vi "Handle Help.vi"(8 "error in (no error)":errorcluster, 10 "Command":variant, 11 "Instrument in":refnum<class "Instrument.lvclass">) -> (0 "error out":errorcluster, 2 "Variant":variant, 3 "Instrument out":refnum<class "Instrument.lvclass">)   [LabVIEW 2019, in "Instrument.lvclass"]
uses:
  Instrument.lvclass
  Typedefs/Instrument.Commands--Enum.ctl
  Typedefs/PrivateEvents--Instrument.DataToLog.ctl
  Typedefs/Instrument.Help--cluster.ctl
  Typedefs/Instrument.API_Help.Param--Cluster.ctl
  5679b731-02d5-469c-8409-12dd10f8f74d.vi
  <vilib>/JDP Science/JSONtext/Variant to JSON Text.vi
  <vilib>/JDP Science/JSONtext/LVClass Serializer/JSONtext LVClass Serializer.lvclass
  <userlib>/LevyLab/JSON-RPC/JSON-RPC.lvlib
  Help/Help.lvclass
  <vilib>/Utility/Data Type/NI_Data Type.lvlib
  <vilib>/JDP Science/JSONtext/JSONtext.lvlib
panel:
  out "<JSON>":string
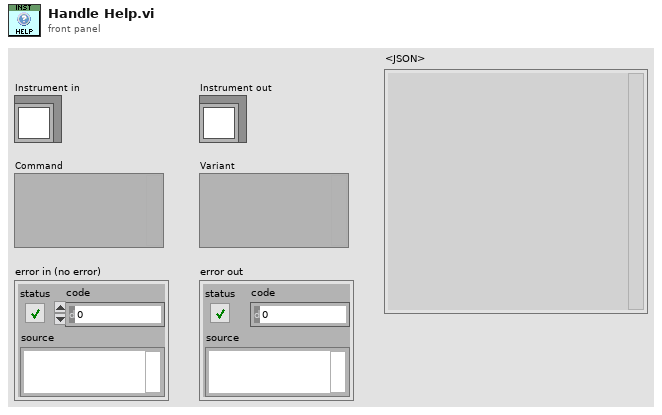
[diagram p1: front panel]
types:
  T1 = typedef "Instrument.lvclass/PrivateEvents--Instrument.DataToLog.ctl" = cluster{"Path(s)":string, "Data":variant}
  T2 = typedef "Instrument.lvclass/Instrument.Commands--Enum.ctl" = enum16{"ACK", "HELP", "setConfiguration", "setLogData", "getAll", "getAllData"}
  T3 = cluster{"number1":dbl, "number2":dbl, "string1":string}
  T4 = typedef "Instrument.lvclass/Instrument.Help--cluster.ctl" = cluster{"description":string, "documentation":string, "example":string}
  T5 = typedef "NI_Data Type.lvlib/Data Type.ctl" = enum8{"Invalid Type", "Void", "I8", "I16", "I32", "I64", "U8", "U16", "U32", "U64", "Single Float", "Double Float", "Extended Float", "Single Complex", "Double Complex", "Extended Complex", "Enum U8", "Enum U16", "Enum U32", "Enum U64", "Single Float With Unit", "Double Float With Unit", "Extended Float With Unit", "Single Complex with Unit", "Double Complex with Unit", "Extended Complex with Unit", "Boolean", "String", "Path", "Picture", "Tag", "Array", "Cluster", "Variant", "LV Variant", "Waveform", "Timestamp", "Digital Waveform", "Digital Data", "ExpressData", "Refnum", "External Data", "VI", "Poly VI", "LabVIEW Class Instance", "Fixed Point", "Set Collection", "Map Collection"}
  T6 = typedef "Instrument.lvclass/Instrument.API_Help.Param--Cluster.ctl" = cluster{"parameter_name":string, "description":string, "min_value":variant, "max_value":variant, "units":string}
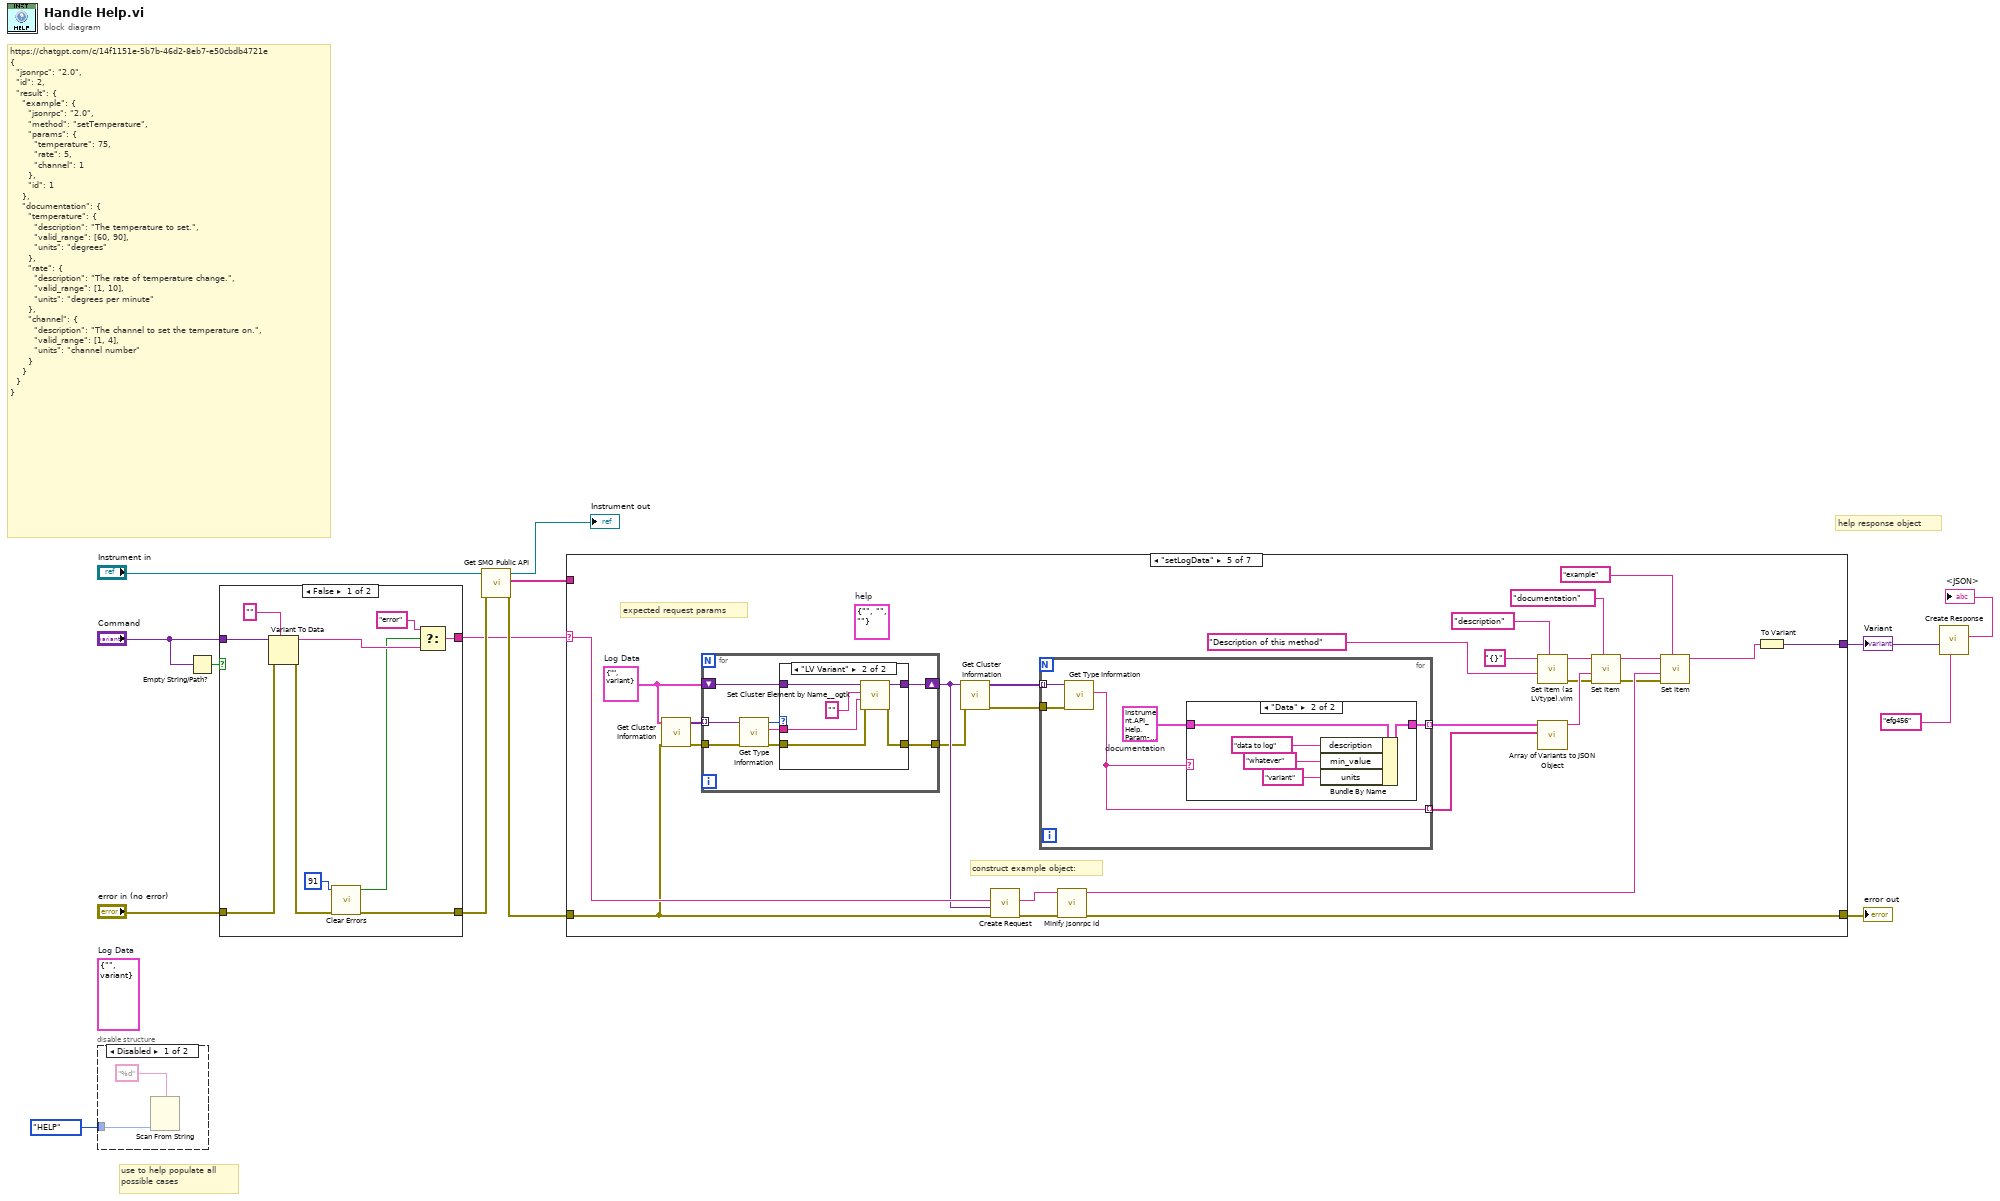
[diagram p0: block diagram]
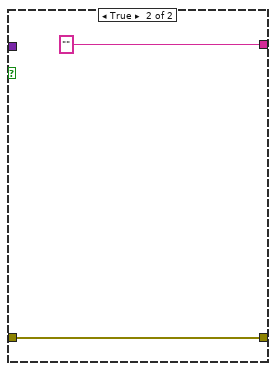
[diagram p2: hidden frame]
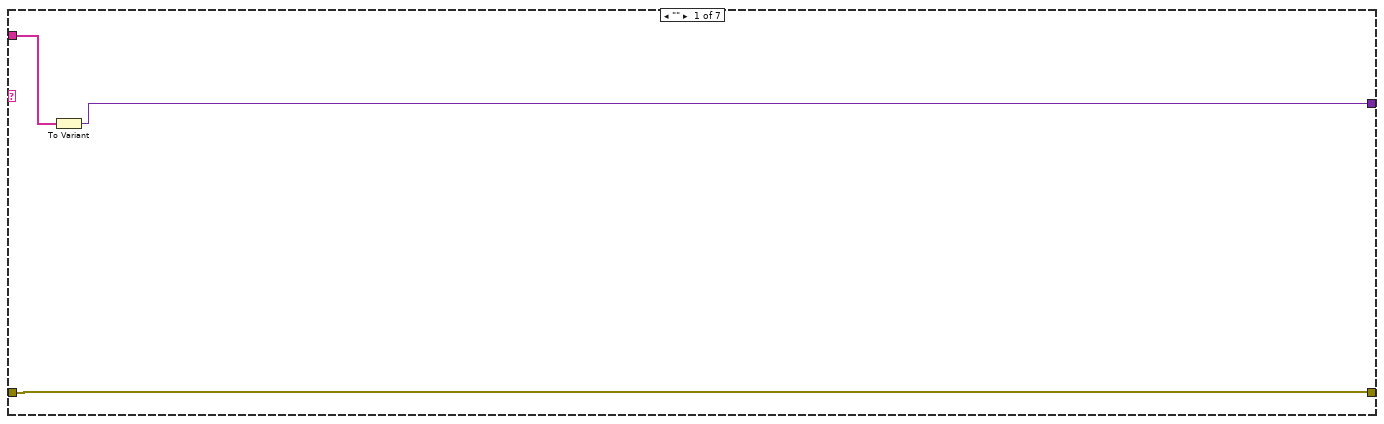
[diagram p4: hidden frame]
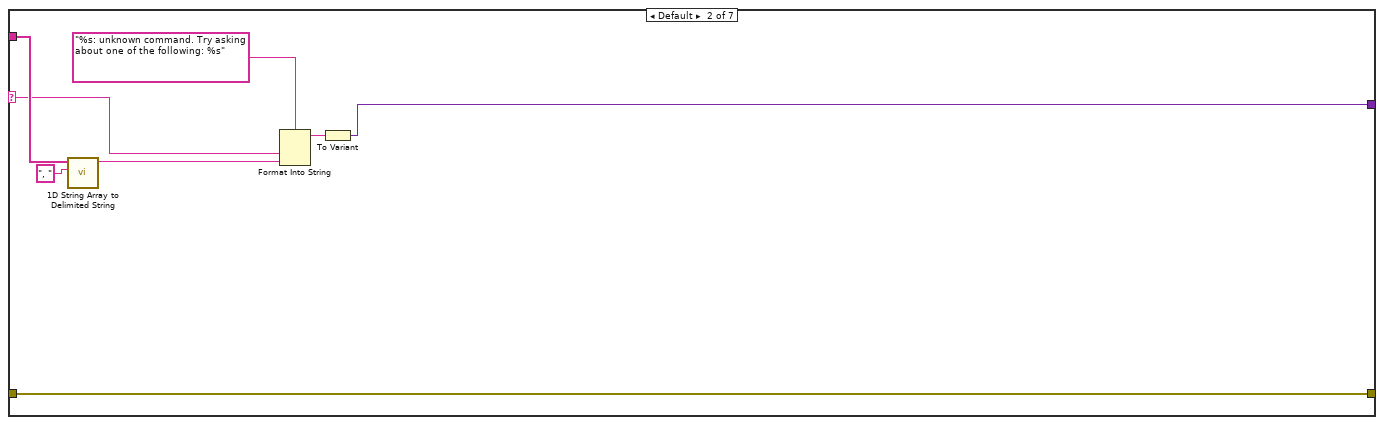
[diagram p5: hidden frame]
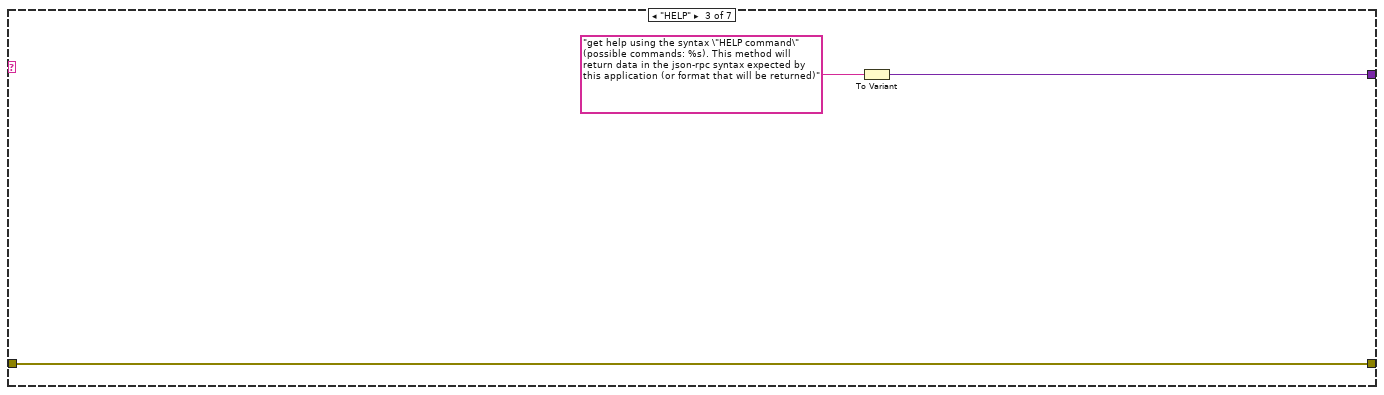
[diagram p6: hidden frame]
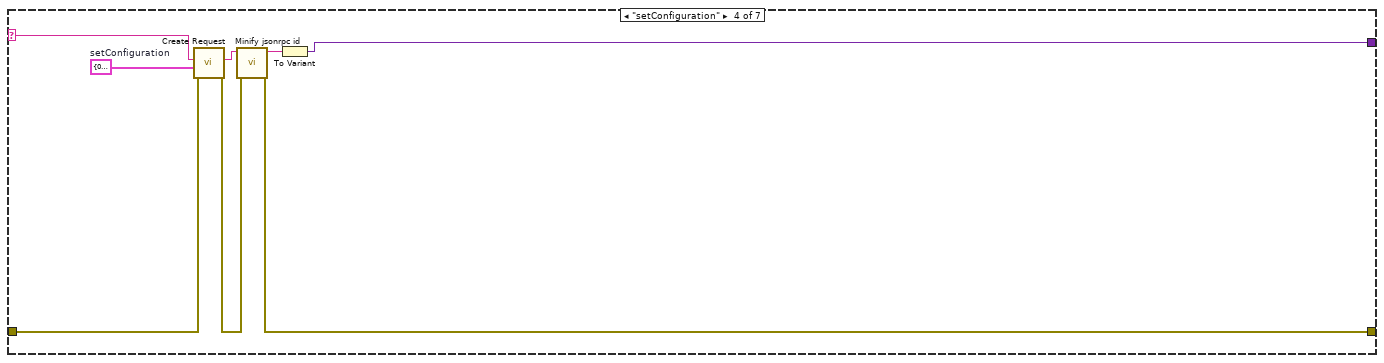
[diagram p7: hidden frame]
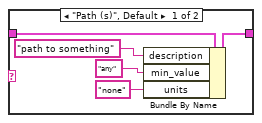
[diagram p9: hidden frame]
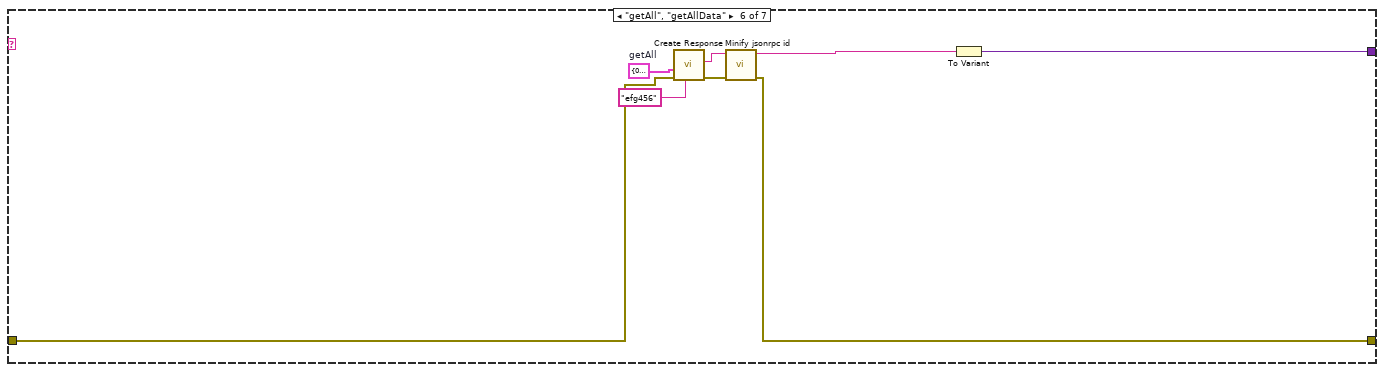
[diagram p10: hidden frame]
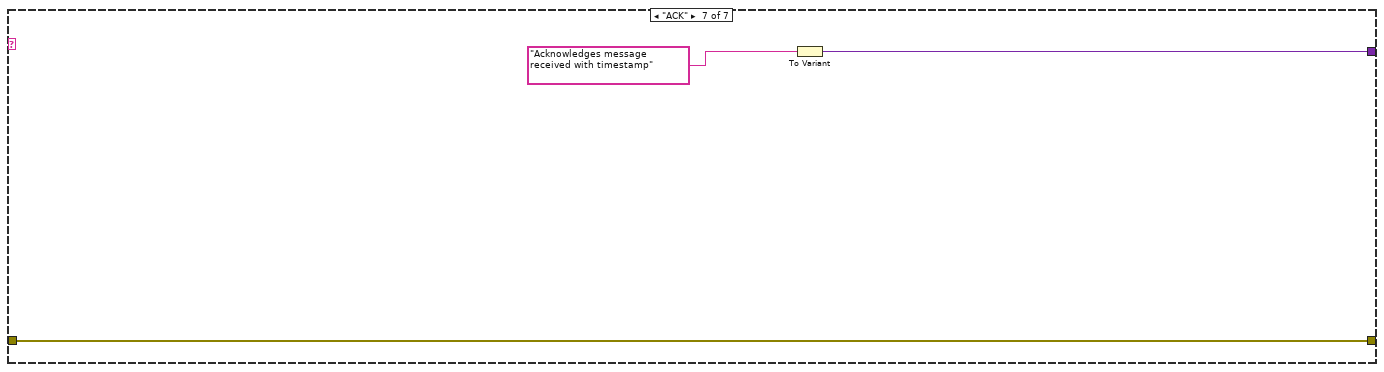
[diagram p11: hidden frame]
diagram:
  (unwired) T1 {"Path(s)"="", "Data"=variant}  # Log Data
  # "help response object"
  # "https://chatgpt.com/c/14f1151e-5b7b-46d2-8eb7-e50cbdb4721e\n{\n  \"jsonrpc\": \"2.0\",\n  \"id\": 2,\n  \"result\": {\n    \"example\": {\n      \"jsonrpc\": \"2.0\",\n      \"method\": \"setTemperature\",\n      \"params\": {\n        \"temperature\": 75,\n        \"rate\": 5,\n        \"channel\": 1\n      },\n      \"id\": 1\n    },\n    \"documentation\": {\n      \"temperature\": {\n        \"description\": \"The temperature to set.\",\n        \"valid_range\": [60, 90],\n        \"units\": \"degrees\"\n      },\n      \"rate\": {\n        \"description\": \"The rate of temperature change.\",\n        \"valid_range\": [1, 10],\n        \"units\": \"degrees per minute\"\n      },\n      \"channel\": {\n        \"description\": \"The channel to set the temperature on.\",\n        \"valid_range\": [1, 4],\n        \"units\": \"channel number\"\n      }\n    }\n  }\n}"
  # "use to help populate all\npossible cases"
  n1 = disable-structure shown="Disabled" {
    disable-tunnel: Instrument.Commands--Enum."HELP" ("Commands") -> [w16 _]
    frame Disabled {
      n2 = Scan From String(format string="%d", default 1=w16) -> (input string=w17:string)  [unwired: 3 in, 3 out]
    }
    frame Enabled {
    }
  }
  n3 = Empty String/Path?(string/path="Command") -> (empty?=w12:bool)
  n4 = case shown="False" w12 {
    tunnel: "error in (no error)" -> [w27 w29]
    tunnel: [w21 ""] -> w2
    tunnel: [w23 w29] -> w4
    tunnel: "Command" -> [w25 _]
    frame False {
      n5 = Variant To Data(error in=w27, type="", Variant=w25) -> (data=w22:string, error out=w24:errorcluster)
      n6 = call <vilib>:"Clear Errors.vi"("error in (no error)"=w24, "specific error code to clear (0: all)"=91) -> ("error out"=w23:errorcluster, "specific error cleared?"=w18:bool)  [unwired: 4 in]
      n7 = Select(t="error", s=w18, f=w22) -> (s? t:f=w21:string)
    }
    frame True {
    }
  }
  n8 = call-dynamic "Get SMO Public API.vi"("error in (no error)"=w4, "Instrument in"="Instrument in") -> ("error out"=w3:errorcluster, "commands"=w10:string[], "Instrument out"=→"Instrument out":refnum<class "Instrument.lvclass">)  [unwired: 7 in]
  n9 = case shown="\"setLogData\"" w2 {
    selector: w2 -> [_ w33 _ w51 w77 _ _]
    tunnel: [w32 w40 w43 w50 w78 w117 w119] -> w8
    tunnel: w3 -> [w30 w35 w42 w44 w52 w112 w118]
    tunnel: [w30 w35 w42 w46 w74 w113 w118] -> w14
    tunnel: w10 -> [w31 w34 _ _ _ _ _]
    frame "" {
      n10 = To Variant(anything=w31) -> (Variant=w32:variant)
    }
    frame Default {
      n11 = call <vilib>:"1D String Array to Delimited String.vi"("delimiter"=", ", "string array"=w34) -> ("delimited string"=w36:string)  [unwired: 9 in]
      n12 = Format Into String(format string="%s: unknown command. Try asking about one of the following: %s", w33, w36) -> (resulting string=w38:string)  [unwired: 2 in, 1 out]
      n13 = To Variant(anything=w38) -> (Variant=w40:variant)
    }
    frame "HELP" {
      n14 = To Variant(anything="get help using the syntax \"HELP command\" (possible commands: %s). This method will return data in the json-rpc syntax expected by this application (or format that will be returned)") -> (Variant=w43:variant)
    }
    frame "setConfiguration" {
      w45 = T3 {"number1"=0.0, "number2"=0.0, "string1"=""}  # setConfiguration
      n15 = call <userlib>:"Create Request.vi"("error in (no error)"=w44, "params"=w45, "method"=w51) -> ("error out"=w47:errorcluster, "<JSON> Requests"=w49:string)  [unwired: 6 in, 1 out]
      n16 = call "Minify jsonrpc id.vi"("error in (no error)"=w47, "<JSON> Requests"=w49) -> ("error out"=w46:errorcluster, "<JSON>"=w48:string)  [unwired: 8 in]
      n17 = To Variant(anything=w48) -> (Variant=w50:variant)
    }
    frame "setLogData" {
      (unwired) T4 {"description"="", "documentation"="", "example"=""}  # help
      w56 = T1 {"Path(s)"="", "Data"=variant}  # Log Data
      # "construct example object:"
      # "expected request params"
      n18 = call <vilib>:"Get Cluster Information.vi"("error in (no error)"=w52, "variant"=w56) -> ("error out"=w55:errorcluster, "cluster elements"=w69:variant[])  [unwired: 8 in]
      n19 = for {
        tunnel: w69 -> [w84] mode=indexing
        shift-right: [w82] -> w68
        shift-left: w56 -> [w83]
        tunnel: w55 -> [w81]
        tunnel: [w79] -> w54
        n20 = call <vilib>:"Get Type Information.vi"("error in (no error)"=w81, "variant"=w84) -> ("error out"=w80:errorcluster, "name"=w86:string, "type"=w85:T5)  [unwired: 5 in, 2 out]
        n21 = case shown="\"LV Variant\"" w85 {
          tunnel: w86 -> [_ w92]
          tunnel: [w88 w94] -> w82
          tunnel: w83 -> [w88 w93]
          tunnel: w80 -> [w87 w90]
          tunnel: [w87 w89] -> w79
          frame Default {
          }
          frame "LV Variant" {
            n22 = call <userlib>:"Set Cluster Element by Name__ogtk.vi"("error in (no error)"=w90, "Element Name (\"\": New Element Data Name)"=w92, "New Element Value"="", "Cluster"=w93) -> ("error out"=w89:errorcluster, "VCluster out"=w94:variant)  [unwired: 5 in, 1 out]
          }
        }
      }
      n23 = call <vilib>:"Get Cluster Information.vi"("error in (no error)"=w54, "variant"=w68) -> ("error out"=w73:errorcluster, "cluster elements"=w72:variant[])  [unwired: 8 in]
      n24 = call <userlib>:"Create Request.vi"("error in (no error)"=w52, "params"=w68, "method"=w77) -> ("error out"=w75:errorcluster, "<JSON> Requests"=w76:string)  [unwired: 6 in, 1 out]
      n25 = for {
        tunnel: w73 -> [w99]
        tunnel: w72 -> [w98] mode=indexing
        tunnel: [w96] -> w71 mode=indexing
        tunnel: [w95] -> w70 mode=indexing
        w97 = T6 {"parameter_name"="", "description"="", "min_value"=variant(string ""), "max_value"=variant(string ""), "units"=""}  # documentation
        n26 = call <vilib>:"Get Type Information.vi"("error in (no error)"=w99, "variant"=w98) -> ("name"=w95:string)  [unwired: 5 in, 4 out]
        n27 = case shown="\"Data\"" w95 {
          tunnel: w97 -> [w104 w109]
          tunnel: [w101 w105] -> w96
          frame "Path (s)", Default {
            n28 = Bundle By Name(cluster=w104, "description"="path to something", "min_value"="any" ("units"), "units"="none") -> (w101:T6)
          }
          frame "Data" {
            n29 = Bundle By Name(cluster=w109, "description"="data to log", "min_value"="whatever" ("units"), "units"="variant") -> (w105:T6)
          }
        }
      }
      n30 = call "Minify jsonrpc id.vi"("error in (no error)"=w75, "<JSON> Requests"=w76) -> ("error out"=w74:errorcluster, "<JSON>"=w61:string)  [unwired: 8 in]
      n31 = call "Set Item (as LVtype).vim"("$Path or Item Name"="description", "Anything"="Description of this method" ("description"), "JSON"="{}") -> ("error out"=w57:errorcluster, "<JSON>"=w64:string)  [unwired: 5 in, 1 out]
      n32 = call <vilib>:"Array of Variants to JSON Object.vi"("Names"=w70, "Array"=w71) -> ("<JSON>"=w60:string)  [unwired: 8 in, 1 out]
      n33 = call <vilib>:"Set Item.vi"("$Path or Item Name"="documentation", "error in (no error)"=w57, "JSON to Insert"=w60, "JSON"=w64) -> ("error out"=w58:errorcluster, "<JSON>"=w62:string)  [unwired: 4 in, 1 out]
      n34 = call <vilib>:"Set Item.vi"("$Path or Item Name"="example", "error in (no error)"=w58, "JSON to Insert"=w61, "JSON"=w62) -> ("<JSON>"=w53:string)  [unwired: 4 in, 2 out]
      n35 = To Variant(anything=w53) -> (Variant=w78:variant)
    }
    frame "getAll", "getAllData" {
      w111 = T3 {"number1"=0.0, "number2"=0.0, "string1"=""}  # getAll
      n36 = call <userlib>:"Create Response.vi"("id"="efg456", "error in (no error)"=w112, "result"=w111) -> ("error out"=w114:errorcluster, "<JSON> Response"=w116:string)  [unwired: 7 in]
      n37 = call "Minify jsonrpc id.vi"("error in (no error)"=w114, "<JSON> Requests"=w116) -> ("error out"=w113:errorcluster, "<JSON>"=w115:string)  [unwired: 8 in]
      n38 = To Variant(anything=w115) -> (Variant=w117:variant)
    }
    frame "ACK" {
      n39 = To Variant(anything="Acknowledges message received with timestamp") -> (Variant=w119:variant)
    }
  }
  "Variant" <- w8
  "error out" <- w14
  n40 = call <userlib>:"Create Response.vi"("id"="efg456", "result"=w8) -> ("<JSON> Response"=→"<JSON>":string)  [unwired: 8 in, 1 out]
